vi "Begin.vi"() -> (0 "error out":errorcluster)   [LabVIEW 2012]
doc: "Called before other user functions, this VI is expected to open initial I/O refnums, load in file data, and do all program initialization. Notice that the <B>error out</B> terminal is simply used for data flow. Wiring it to other structures or subVIs ensures that this VI runs first."
uses:
  <vilib>/Rock Robotics/WPI/DriverStation/WPI_DriverStationRobotMode2.ctl
  <vilib>/Rock Robotics/WPI/Joystick/WPI_JoystickDeviceEnum.ctl
  <vilib>/Rock Robotics/WPI/Solenoid/WPI_SolenoidChannel.ctl
  <vilib>/Rock Robotics/SystemInterfaces/DIO/FPGA_DIORelayChannel.ctl
  <vilib>/Rock Robotics/WPI/Relay/WPI_RelayDirection.ctl
  <vilib>/Rock Robotics/SystemInterfaces/DIO/FPGA_DIOChannel.ctl
  <vilib>/Rock Robotics/WPI/Encoder/WPI_EncoderType.ctl
  <vilib>/Rock Robotics/SystemInterfaces/DIO/FPGA_DIOPWMChannel.ctl
  <vilib>/Rock Robotics/SystemInterfaces/AI/FPGA_AIGyroChannel.ctl
  <vilib>/Rock Robotics/SystemInterfaces/Typedef/FPGA_TypedefSolenoidModule.ctl
  Robot Global Data.vi
  <vilib>/Rock Robotics/WPI/Solenoid/WPI_SolenoidOpenSingle.vi
  <vilib>/Rock Robotics/WPI/Solenoid/Deprecated/WPI_SolenoidSetBool.vi
  <vilib>/Rock Robotics/WPI/Counter/WPI_CounterDigitalInputToDigitalSource.vi
  <vilib>/Rock Robotics/WPI/MotorControl/WPI_MotorControlOpen Jaguar.vi
  <vilib>/Rock Robotics/WPI/MotorControl/WPI_MotorControlOpen Victor.vi
  <vilib>/Rock Robotics/WPI/MotorControl/WPI_MotorControlOpen Talon.vi
  <vilib>/Rock Robotics/WPI/RobotDrive/WPI_RobotDriveOpen4MotorWithExistingMotors.vi
  <vilib>/Rock Robotics/WPI/Compressor/WPI_CompressorGetSetRefNum.vi
  <vilib>/Rock Robotics/SystemInterfaces/Typedef/FPGA_TypedefDigitalModule.ctl
  <vilib>/Rock Robotics/WPI/RobotDrive/WPI_RobotDriveOpen4MotorWithTalon.vi
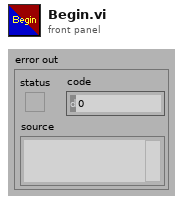
[diagram p1: front panel]
types:
  T1 = typedef "FPGA_DIOChannel.ctl" = enum8{"DIO 1", "DIO 2", "DIO 3", "DIO 4", "DIO 5", "DIO 6", "DIO 7", "DIO 8", "DIO 9", "DIO 10", "DIO 11", "DIO 12", "DIO 13", "DIO 14", "Invalid"}
  T2 = typedef "WPI_SolenoidChannel.ctl" = enum8{"Solenoid 1", "Solenoid 2", "Solenoid 3", "Solenoid 4", "Solenoid 5", "Solenoid 6", "Solenoid 7", "Solenoid 8", "Invalid"}
  T3 = typedef "FPGA_TypedefSolenoidModule.ctl" = enum16{"Solenoid Module 1", "Solenoid Module 2"}
  T4 = typedef "FPGA_AIGyroChannel.ctl" = enum8{"AI 1", "AI 2", "Invalid"}
  T5 = typedef "WPI_EncoderType.ctl" = enum16{"1x", "2x", "4x"}
  T6 = typedef "FPGA_DIORelayChannel.ctl" = enum8{"Relay 1", "Relay 2", "Relay 3", "Relay 4", "Relay 5", "Relay 6", "Relay 7", "Relay 8", "Invalid"}
  T7 = typedef "WPI_JoystickDeviceEnum.ctl" = enum16{"USB 1", "USB 2", "USB 3", "USB 4", "Kinect 1", "Kinect 2"}
  T8 = typedef "FPGA_DIOPWMChannel.ctl" = enum8{"PWM 1", "PWM 2", "PWM 3", "PWM 4", "PWM 5", "PWM 6", "PWM 7", "PWM 8", "PWM 9", "PWM 10", "Invalid"}
  T9 = typedef "WPI_RelayDirection.ctl" = enum16{"Both directions", "Forward only", "Reverse only"}
  T10 = typedef "WPI_DriverStationRobotMode2.ctl" = enum16{"Autonomous Disabled", "Autonomous Enabled", "Teleop Disabled", "Teleop Enabled", "Timeout", "Finish", "Test Disabled", "Test Enabled"}
  T11 = typedef "WPI_RobotDriveDevRef.ctl" = cluster{"DevStatus":errorcluster, "Motors[]":T12[], "Square Inputs":bool, "Max Output":dbl, "Isochronous":bool}
  T12 = typedef "WPI_MotorControlDeviceRef.ctl" = cluster{"DeviceStatus":errorcluster, "Type":enum16{"PWM", "CAN"}, "PWM":cluster{"Digital Module":T13, "PWM Channel":T8, "DeadBand":T14}, "CAN":cluster{"Device Number":u8, "Control Mode":T15, "Semaphore":T16, "Max Vout":dbl}, "Invert":bool, "TransformRef":T17, "InvTransformRef":T17}
  T13 = typedef "FPGA_TypedefDigitalModule.ctl" = enum16{"Digital Module 1", "Digital Module 2"}
  T14 = typedef "WPI_PWMDeadband.ctl" = cluster{"Name":string, "maxPositivePwm":i32, "minPositivePwm":i32, "centerPwm":i32, "maxNegativePwm":i32, "minNegativePwm":i32, "angularRange":u16}
  T15 = typedef "WPI_CANJaguar_ControlMode.ctl" = enum8{"Percent VBus", "Current", "Speed", "Position", "Voltage"}
  T16 = typedef "Semaphore RefNum" = refnum<k1>
  T17 = typedef "WPI_PWMTransform_ConPane.ctl" = refnum<vi>
  T18 = typedef "WPI_DigitalInputDevRef.ctl" = cluster{"DevStatus":errorcluster, "DIO Channel":T1, "Digital Module":T13}
  T19 = typedef "WPI_ServoDeviceRef.ctl" = cluster{"DeviceStatus":errorcluster, "Digital Module":T13, "PWM Channel":T8, "DeadBand":T14}
  T20 = typedef "WPI_CompressorDevRef.ctl" = cluster{"DevStatus":errorcluster, "DigitalInputDevRef":T18, "RelayDevRef":T21}
  T21 = typedef "WPI_RelayDevRef.ctl" = cluster{"DevStatus":errorcluster, "Relay Channel":T6, "Digital Module":T13, "Relay Direction":T9}
  T22 = typedef "WPI_JoystickDevRef.ctl" = cluster{"Device":T7}
  T23 = typedef "WPI_SolenoidDevRef.ctl" = cluster{"DevStatus":errorcluster, "Solenoid Module":T3, "Forward Solenoid Channel":T2, "Reverse Solenoid Channel":T2}
  T24 = typedef "FPGA_CounterEncoderSourceConvertionLVSourceType.ctl" = cluster{"DevStatus":errorcluster, "AnalogTriggerMode?":bool, "DigitalMode":cluster{"Digital Module":T13, "DIO Channel":T25}, "AnalogTriggerMode":cluster{"AnalogTriggerIndex":T26, "OutputType":T27}}
  T25 = typedef "FPGA_DIODigitalSourceChannel.ctl" = enum8{"DIO 1", "DIO 2", "DIO 3", "DIO 4", "DIO 5", "DIO 6", "DIO 7", "DIO 8", "DIO 9", "DIO 10", "DIO 11", "DIO 12", "DIO 13", "DIO 14", "Disabled"}
  T26 = typedef "FPGA_AnalogTriggerIndex.ctl" = enum8{"Trig 0", "Trig 1", "Trig 2", "Trig 3", "Trig 4", "Trig 5", "Trig 6", "Trig 7", "Invalid"}
  T27 = typedef "FPGA_AnalogTriggerOutType.ctl" = enum16{"InWindow", "TriggerState", "Rising", "Falling"}
  T28 = typedef "WPI_GyroDevRef.ctl" = cluster{"DevStatus":errorcluster, "Analog Module":T29, "Analog Channel":T30, "Offset":dbl, "Gain (VoltsPerDegree/Second)":dbl}
  T29 = typedef "FPGA_TypedefAnalogModule.ctl" = enum16{"Analog Module 1", "Analog Module 2"}
  T30 = typedef "FPGA_AIChannel.ctl" = enum8{"AI 1", "AI 2", "AI 3", "AI 4", "AI 5", "AI 6", "AI 7", "AI 8", "Invalid"}
  T31 = typedef "WPI_EncoderDevRef.ctl" = cluster{"DevStatus":errorcluster, "EncoderIndex":T32, "CounterIndex":T33, "DistancePerCount":dbl, "Decoding Type":T5}
  T32 = typedef "FPGA_EncoderIdx.ctl" = enum8{"Enc 0", "Enc 1", "Enc 2", "Enc 3", "Invalid"}
  T33 = typedef "FPGA_CounterCtrSystemIndex.ctl" = enum8{"Ctr 0", "Ctr 1", "Ctr 2", "Ctr 3", "Ctr 4", "Ctr 5", "Ctr 6", "Ctr 7", "Invalid"}
  T34 = cluster{"Target Voltage":dbl, "Target Speed":dbl, "Angle Up?":bool}
  T35 = cluster{"Target Voltage":dbl, "Target Speed":i32, "Angle Up?":bool}
  T36 = cluster{"Target Voltage":i32, "Target Speed":i32, "Angle Up?":bool}
  T37 = cluster{"Target Voltage":dbl, "Target Speed":i32, "Angle Up?":bool}[]
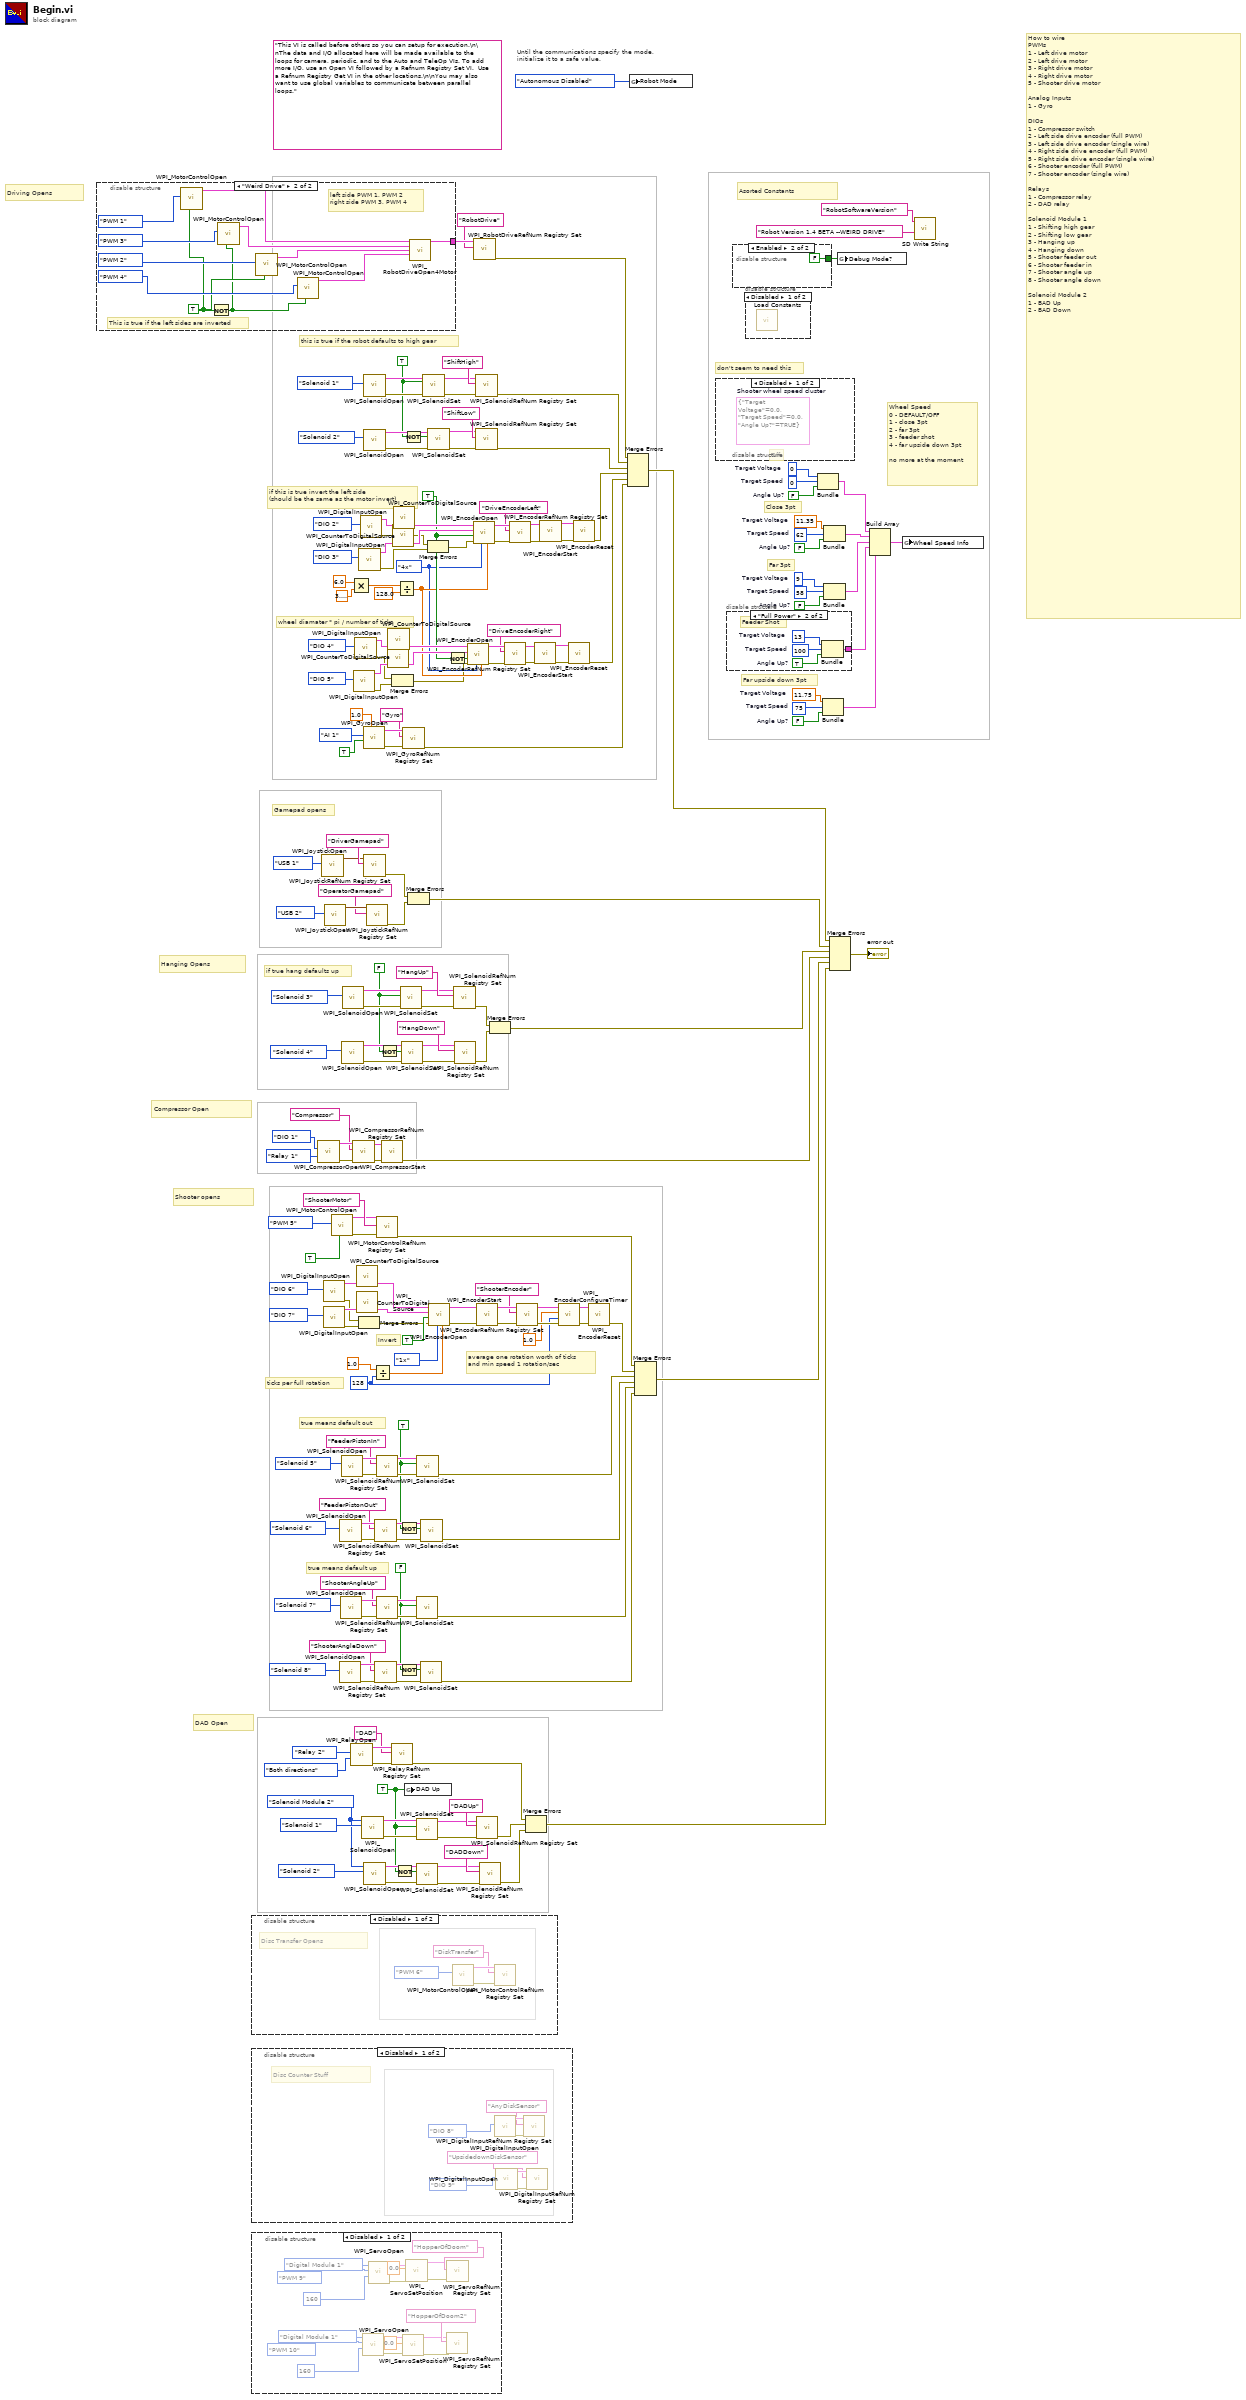
[diagram p0: block diagram]
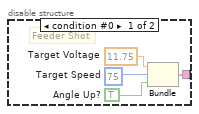
[diagram p3: hidden frame]
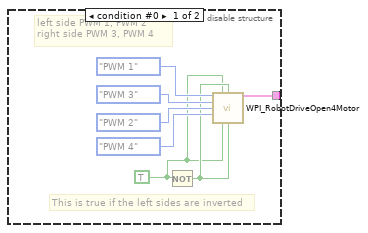
[diagram p4: hidden frame]
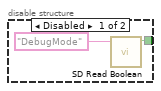
[diagram p5: hidden frame]
diagram:
  w3 = FALSE  # Angle Up?
  w2 = 58  # Target Speed
  w1 = 9  # Target Voltage
  w7 = FALSE  # Angle Up?
  w6 = 75  # Target Speed
  w5 = 11.75  # Target Voltage
  w11 = FALSE  # Angle Up?
  w10 = 0  # Target Speed
  w9 = 0  # Target Voltage
  w13 = u8 128 ("Number Samples to Average")
  w20 = FALSE  # Angle Up?
  w21 = 62  # Target Speed
  w22 = 11.35  # Target Voltage
  w82 = FALSE
  w96 = TRUE
  w57 = TRUE
  w59 = FPGA_TypedefSolenoidModule."Solenoid Module 2" ("Solenoid Module (Module 1)")
  w60 = FALSE
  w62 = WPI_EncoderType."4x" ("Decoding Type")
  w64 = TRUE ("Invert Direction (False)")
  w80 = TRUE
  (unwired) "This VI is called before others so you can setup for execution.\n\nThe data and I/O allocated here will be made available to the loops for camera, periodic, and to the Auto and TeleOp VIs. To add more I/O, use an Open VI followed by a Refnum Registry Set VI.  Use a Refnum Registry Get VI in the other locations.\n\nYou may also want to use global variables to communicate between parallel loops."
  # "don't seem to need this"
  # "Far 3pt"
  # "Far upside down 3pt"
  # "average one rotation worth of ticks\nand min speed 1 rotation/sec"
  # "Close 3pt"
  # "How to wire\nPWMs\n1 - Left drive motor\n2 - Left drive motor\n3 - Right drive motor\n4 - Right drive motor\n5 - Shooter drive motor\n\nAnalog Inputs\n1 - Gyro\n\nDIOs\n1 - Compressor switch\n2 - Left side drive encoder (full PWM)\n3 - Left side drive encoder (single wire)\n4 - Right side drive encoder (full PWM)\n5 - Right side drive encoder (single wire)\n6 - Shooter encoder (full PWM)\n7 - Shooter encoder (single wire)\n\nRelays\n1 - Compressor relay\n2 - DAD relay\n\nSolenoid Module 1\n1 - Shifting high gear\n2 - Shifting low gear\n3 - Hanging up\n4 - Hanging down\n5 - Shooter feeder out\n6 - Shooter feeder in\n7 - Shooter angle up\n8 - Shooter angle down\n\nSolenoid Module 2\n1 - BAD Up\n2 - BAD Down"
  # "Asorted Constants"
  # "true means default up"
  # "true means default out"
  # "if true hang defaults up"
  # "Gamepad opens"
  # "wheel diamater * pi / number of ticks"
  # "if this is true invert the left side\n(should be the same as the motor invert)"
  # "this is true if the robot defaults to high gear"
  # "Compressor Open"
  # "Wheel Speed\n0 - DEFAULT/OFF\n1 - close 3pt\n2 - far 3pt\n3 - feeder shot\n4 - far upside down 3pt\n\nno more at the moment"
  # "DAD Open"
  # "Hanging Opens"
  # "Driving Opens"
  # "Shooter opens"
  # "Invert"
  # "ticks per full rotation"
  # "Until the communications specify the mode,\ninitialize it to a safe value."
  n1 = disable-structure shown="\"Weird Drive\"" {
    disable-tunnel: [w217 w232] -> w210
    frame condition #0 {
      w215 = TRUE ("Rear Left Motor Inverted")
      # "left side PWM 1, PWM 2\nright side PWM 3, PWM 4"
      # "This is true if the left sides are inverted"
      n2 = Not(x=w215) -> (.not. x?=w216:bool)
      n3 = call-poly <vilib>:"WPI_RobotDriveOpen4Motor.vi"("Rear Left Motor"=FPGA_DIOPWMChannel."PWM 1", "Rear Left Motor Inverted"=w215, "Rear Right Motor Inverted"=w216, "Rear Right Motor"=FPGA_DIOPWMChannel."PWM 3", "Front Left Motor"=FPGA_DIOPWMChannel."PWM 2", "Front Right Motor"=FPGA_DIOPWMChannel."PWM 4" ("Front Left Motor"), "Front Left Motor Inverted"=w215, "Front Right Motor Inverted"=w216) -> ("RobotDriveDevRef"=w217:T11)  [unwired: 6 in, 1 out]
    }
    frame condition #1 (active) {
      w227 = TRUE ("Rear Left Motor Inverted")
      # "left side PWM 1, PWM 2\nright side PWM 3, PWM 4"
      # "This is true if the left sides are inverted"
      n4 = call-poly <vilib>:"WPI_MotorControlOpen.vi"("Invert"=w227, "PWM Channel"=FPGA_DIOPWMChannel."PWM 1" ("Rear Left Motor")) -> ("MotorControlDeviceRef"=w225:T12)  [unwired: 8 in, 1 out]
      n5 = Not(x=w227) -> (.not. x?=w226:bool)
      n6 = call-poly <vilib>:"WPI_MotorControlOpen.vi"("Invert"=w226, "PWM Channel"=FPGA_DIOPWMChannel."PWM 3" ("Rear Right Motor")) -> ("MotorControlDeviceRef"=w224:T12)  [unwired: 8 in, 1 out]
      n7 = call-poly <vilib>:"WPI_MotorControlOpen.vi"("Invert"=w227, "PWM Channel"=FPGA_DIOPWMChannel."PWM 2" ("Front Left Motor")) -> ("MotorControlDeviceRef"=w223:T12)  [unwired: 8 in, 1 out]
      n8 = call-poly <vilib>:"WPI_MotorControlOpen.vi"("Invert"=w226, "PWM Channel"=FPGA_DIOPWMChannel."PWM 4" ("Front Left Motor")) -> ("MotorControlDeviceRef"=w222:T12)  [unwired: 8 in, 1 out]
      n9 = call-poly <vilib>:"WPI_RobotDriveOpen4Motor.vi"("Rear Left Motor Dev Ref"=w225, "Rear Right Motor Dev Ref"=w224, "Front Left Motor Dev Ref"=w223, "Front Right Motor Dev Ref"=w222) -> ("RobotDriveDevRef"=w232:T11)  [unwired: 10 in, 1 out]
    }
  }
  n10 = disable-structure shown="Disabled" {
    frame Disabled {
      # "Disc Transfer Opens"
      n11 = call-poly <vilib>:"WPI_MotorControlOpen.vi"("PWM Channel"=FPGA_DIOPWMChannel."PWM 6") -> ("error out"=w234:errorcluster, "MotorControlDeviceRef"=w235:T12)  [unwired: 9 in]
      n12 = call <vilib>:"WPI_MotorControlRefNum Registry Set.vi"("error in (no error)"=w234, "refnum name"="DiskTransfer", "MotorControlDevRef"=w235) -> ()  [unwired: 7 in, 2 out]
    }
    frame Enabled {
    }
  }
  n13 = disable-structure shown="Disabled" {
    frame Disabled {
      # "Disc Counter Stuff"
      n14 = call <vilib>:"WPI_DigitalInputOpen.vi"("DIO Channel"=FPGA_DIOChannel."DIO 8") -> ("error out"=w244:errorcluster, "DigitalInputDevRef"=w243:T18)  [unwired: 9 in]
      n15 = call <vilib>:"WPI_DigitalInputOpen.vi"("DIO Channel"=FPGA_DIOChannel."DIO 9") -> ("error out"=w242:errorcluster, "DigitalInputDevRef"=w241:T18)  [unwired: 9 in]
      n16 = call <vilib>:"WPI_DigitalInputRefNum Registry Set.vi"("error in (no error)"=w244, "refnum name"="AnyDiskSensor", "DigitalInputDevRef"=w243) -> ()  [unwired: 7 in, 2 out]
      n17 = call <vilib>:"WPI_DigitalInputRefNum Registry Set.vi"("error in (no error)"=w242, "refnum name"="UpsidedownDiskSensor", "DigitalInputDevRef"=w241) -> ()  [unwired: 7 in, 2 out]
    }
    frame Enabled {
    }
  }
  n18 = disable-structure shown="Disabled" {
    frame Disabled {
      n19 = call <vilib>:"WPI_ServoOpen.vi"("Angular Range"=160, "PWM Channel"=FPGA_DIOPWMChannel."PWM 10", "Digital Module (Module 1)"=FPGA_TypedefDigitalModule."Digital Module 1") -> ("error out"=w250:errorcluster, "ServoDeviceRef"=w249:T19)  [unwired: 7 in]
      n20 = call <vilib>:"WPI_ServoOpen.vi"("Angular Range"=160, "PWM Channel"=FPGA_DIOPWMChannel."PWM 9", "Digital Module (Module 1)"=FPGA_TypedefDigitalModule."Digital Module 1") -> ("error out"=w254:errorcluster, "ServoDeviceRef"=w253:T19)  [unwired: 7 in]
      n21 = call <vilib>:"WPI_ServoSetPosition.vi"("error in (no error)"=w250, "Position"=0.0, "ServoDeviceRef"=w249) -> ("error out"=w247:errorcluster, "ServoDeviceRef"=w248:T19)  [unwired: 7 in]
      n22 = call <vilib>:"WPI_ServoSetPosition.vi"("error in (no error)"=w254, "Position"=0.0, "ServoDeviceRef"=w253) -> ("error out"=w252:errorcluster, "ServoDeviceRef"=w251:T19)  [unwired: 7 in]
      n23 = call <vilib>:"WPI_ServoRefNum Registry Set.vi"("error in (no error)"=w247, "refnum name"="HopperOfDoom2", "ServoDeviceRef"=w248) -> ()  [unwired: 7 in, 2 out]
      n24 = call <vilib>:"WPI_ServoRefNum Registry Set.vi"("error in (no error)"=w252, "refnum name"="HopperOfDoom", "ServoDeviceRef"=w251) -> ()  [unwired: 7 in, 2 out]
    }
    frame Enabled {
    }
  }
  n25 = call <vilib>:"WPI_CompressorOpen.vi"("Pressure Switch DIO Channel"=FPGA_DIOChannel."DIO 1", "Relay Channel"=FPGA_DIORelayChannel."Relay 1") -> ("CompressorDevRef"=w162:T20, "error out"=w160:errorcluster)  [unwired: 12 in]
  n26 = call <vilib>:"WPI_JoystickOpen.vi"("JoystickDevice"=WPI_JoystickDeviceEnum."USB 1") -> ("JoystickDevRef"=w212:T22)  [unwired: 10 in]
  n27 = call <vilib>:"WPI_DigitalInputOpen.vi"("DIO Channel"=FPGA_DIOChannel."DIO 6") -> ("error out"=w178:errorcluster, "DigitalInputDevRef"=w191:T18)  [unwired: 9 in]
  n28 = call <vilib>:"WPI_DigitalInputOpen.vi"("DIO Channel"=FPGA_DIOChannel."DIO 7") -> ("error out"=w177:errorcluster, "DigitalInputDevRef"=w187:T18)  [unwired: 9 in]
  n29 = call <vilib>:"WPI_JoystickOpen.vi"("JoystickDevice"=WPI_JoystickDeviceEnum."USB 2") -> ("JoystickDevRef"=w164:T22)  [unwired: 10 in]
  n30 = call-poly <vilib>:"WPI_MotorControlOpen.vi"("Invert"=TRUE, "PWM Channel"=FPGA_DIOPWMChannel."PWM 5") -> ("error out"=w171:errorcluster, "MotorControlDeviceRef"=w172:T12)  [unwired: 8 in]
  n31 = call-poly <vilib>:"WPI_SolenoidOpen.vi"("Solenoid Channel"=WPI_SolenoidChannel."Solenoid 8") -> ("error out"=w92:errorcluster, "SolenoidDevRef"=w91:T23)  [unwired: 9 in]
  n32 = call-poly <vilib>:"WPI_SolenoidOpen.vi"("Solenoid Channel"=WPI_SolenoidChannel."Solenoid 6") -> ("error out"=w106:errorcluster, "SolenoidDevRef"=w105:T23)  [unwired: 9 in]
  n33 = call-poly <vilib>:"WPI_SolenoidOpen.vi"("Solenoid Channel"=WPI_SolenoidChannel."Solenoid 7") -> ("error out"=w87:errorcluster, "SolenoidDevRef"=w88:T23)  [unwired: 9 in]
  n34 = call-poly <vilib>:"WPI_SolenoidOpen.vi"("Solenoid Channel"=WPI_SolenoidChannel."Solenoid 5") -> ("error out"=w101:errorcluster, "SolenoidDevRef"=w102:T23)  [unwired: 9 in]
  n35 = call-poly <vilib>:"WPI_SolenoidOpen.vi"("Solenoid Channel"=WPI_SolenoidChannel."Solenoid 4") -> ("error out"=w128:errorcluster, "SolenoidDevRef"=w129:T23)  [unwired: 9 in]
  n36 = call-poly <vilib>:"WPI_SolenoidOpen.vi"("Solenoid Channel"=WPI_SolenoidChannel."Solenoid 3") -> ("error out"=w131:errorcluster, "SolenoidDevRef"=w130:T23)  [unwired: 9 in]
  n37 = Multiply(x=6.0, y=3.141592653589793) -> (x*y=w149:dbl)
  n38 = call <vilib>:"WPI_RelayOpen.vi"("Relay Direction"=WPI_RelayDirection."Both directions", "Relay Channel"=FPGA_DIORelayChannel."Relay 2") -> ("error out"=w194:errorcluster, "RelayDevRef"=w193:T21)  [unwired: 8 in]
  n39 = call <vilib>:"WPI_CompressorRefNum Registry Set.vi"("error in (no error)"=w160, "refnum name"="Compressor", "CompressorDevRef"=w162) -> ("error out"=w110:errorcluster, "CompressorDevRef"=w111:T20)  [unwired: 7 in]
  n40 = call <vilib>:"WPI_DigitalInputOpen.vi"("DIO Channel"=FPGA_DIOChannel."DIO 5") -> ("error out"=w50:errorcluster, "DigitalInputDevRef"=w72:T18)  [unwired: 9 in]
  n41 = call <vilib>:"WPI_DigitalInputOpen.vi"("DIO Channel"=FPGA_DIOChannel."DIO 4") -> ("error out"=w49:errorcluster, "DigitalInputDevRef"=w71:T18)  [unwired: 9 in]
  n42 = call-poly <vilib>:"WPI_CounterToDigitalSource.vi"("DigitalInputDevRef"=w191) -> ("Digital Source"=w190:T24)  [unwired: 6 in]
  n43 = call-poly <vilib>:"WPI_CounterToDigitalSource.vi"("DigitalInputDevRef"=w187) -> ("Digital Source"=w184:T24)  [unwired: 6 in]
  n44 = Merge Errors(w178, w177) -> (w179:errorcluster)
  n45 = call <vilib>:"WPI_DigitalInputOpen.vi"("DIO Channel"=FPGA_DIOChannel."DIO 3") -> ("error out"=w45:errorcluster, "DigitalInputDevRef"=w152:T18)  [unwired: 9 in]
  n46 = call <vilib>:"WPI_DigitalInputOpen.vi"("DIO Channel"=FPGA_DIOChannel."DIO 2") -> ("error out"=w46:errorcluster, "DigitalInputDevRef"=w153:T18)  [unwired: 9 in]
  n47 = call-poly <vilib>:"WPI_SolenoidOpen.vi"("Solenoid Channel"=WPI_SolenoidChannel."Solenoid 1", "Solenoid Module (Module 1)"=w59) -> ("error out"=w115:errorcluster, "SolenoidDevRef"=w119:T23)  [unwired: 8 in]
  n48 = call <vilib>:"WPI_GyroOpen.vi"("Calibration Time (s)"=1.0, "Calibrate On Open"=TRUE, "Analog Channel"=FPGA_AIGyroChannel."AI 1") -> ("error out"=w141:errorcluster, "GyroDevRef"=w140:T28)  [unwired: 6 in, 1 out]
  n49 = call-poly <vilib>:"WPI_SolenoidOpen.vi"("Solenoid Channel"=WPI_SolenoidChannel."Solenoid 1") -> ("error out"=w201:errorcluster, "SolenoidDevRef"=w204:T23)  [unwired: 9 in]
  n50 = call-poly <vilib>:"WPI_SolenoidOpen.vi"("Solenoid Channel"=WPI_SolenoidChannel."Solenoid 2") -> ("error out"=w198:errorcluster, "SolenoidDevRef"=w200:T23)  [unwired: 9 in]
  n51 = call <vilib>:"WPI_JoystickRefNum Registry Set.vi"("refnum name"="DriverGamepad", "JoystickDevRef"=w212) -> ("error out"=w42:errorcluster)  [unwired: 8 in, 1 out]
  n52 = call-poly <vilib>:"WPI_SolenoidOpen.vi"("Solenoid Channel"=WPI_SolenoidChannel."Solenoid 2", "Solenoid Module (Module 1)"=w59) -> ("error out"=w112:errorcluster, "SolenoidDevRef"=w117:T23)  [unwired: 8 in]
  n53 = call <vilib>:"WPI_JoystickRefNum Registry Set.vi"("refnum name"="OperatorGamepad", "JoystickDevRef"=w164) -> ("error out"=w41:errorcluster)  [unwired: 8 in, 1 out]
  n54 = Divide(x=1.0, y=w13) -> (x/y=w14:dbl)
  n55 = call <vilib>:"WPI_SolenoidRefNum Registry Set.vi"("error in (no error)"=w106, "refnum name"="FeederPistonOut", "SolenoidDevRef"=w105) -> ("error out"=w108:errorcluster, "SolenoidDevRef"=w107:T23)  [unwired: 7 in]
  n56 = call <vilib>:"WPI_SolenoidRefNum Registry Set.vi"("error in (no error)"=w92, "refnum name"="ShooterAngleDown", "SolenoidDevRef"=w91) -> ("error out"=w94:errorcluster, "SolenoidDevRef"=w93:T23)  [unwired: 7 in]
  n57 = call <vilib>:"WPI_MotorControlRefNum Registry Set.vi"("error in (no error)"=w171, "refnum name"="ShooterMotor", "MotorControlDevRef"=w172) -> ("error out"=w38:errorcluster)  [unwired: 7 in, 1 out]
  n58 = call <vilib>:"WPI_SolenoidRefNum Registry Set.vi"("error in (no error)"=w101, "refnum name"="FeederPistonIn", "SolenoidDevRef"=w102) -> ("error out"=w99:errorcluster, "SolenoidDevRef"=w100:T23)  [unwired: 7 in]
  n59 = call <vilib>:"WPI_SolenoidRefNum Registry Set.vi"("error in (no error)"=w87, "refnum name"="ShooterAngleUp", "SolenoidDevRef"=w88) -> ("error out"=w85:errorcluster, "SolenoidDevRef"=w86:T23)  [unwired: 7 in]
  n60 = Not(x=w60) -> (.not. x?=w61:bool)
  n61 = call <vilib>:"WPI_CompressorStart.vi"("error in (no error)"=w110, "CompressorDevRef"=w111) -> ("error out"=w26:errorcluster)  [unwired: 8 in, 1 out]
  n62 = call-poly <vilib>:"WPI_CounterToDigitalSource.vi"("DigitalInputDevRef"=w72) -> ("Digital Source"=w69:T24)  [unwired: 6 in]
  n63 = call-poly <vilib>:"WPI_CounterToDigitalSource.vi"("DigitalInputDevRef"=w71) -> ("Digital Source"=w67:T24)  [unwired: 6 in]
  n64 = call <vilib>:"WPI_RelayRefNum Registry Set.vi"("error in (no error)"=w194, "refnum name"="DAD", "RelayDevRef"=w193) -> ("error out"=w32:errorcluster)  [unwired: 7 in, 1 out]
  n65 = Merge Errors(w49, w50) -> (w48:errorcluster)
  n66 = call-poly <vilib>:"WPI_CounterToDigitalSource.vi"("DigitalInputDevRef"=w152) -> ("Digital Source"=w155:T24)  [unwired: 6 in]
  n67 = call-poly <vilib>:"WPI_CounterToDigitalSource.vi"("DigitalInputDevRef"=w153) -> ("Digital Source"=w157:T24)  [unwired: 6 in]
  n68 = Not(x=w57) -> (.not. x?=w58:bool)
  n69 = Divide(x=w149, y=128.0 ("x")) -> (x/y=w63:dbl)
  n70 = Not(x=w82) -> (.not. x?=w95:bool)
  n71 = Not(x=w96) -> (.not. x?=w109:bool)
  n72 = call-poly <vilib>:"WPI_SolenoidSet.vi"("error in (no error)"=w131, "Value"=w60, "SolenoidDevRef"=w130) -> ("error out"=w124:errorcluster, "SolenoidDevRef"=w127:T23)  [unwired: 7 in]
  n73 = call-poly <vilib>:"WPI_SolenoidSet.vi"("error in (no error)"=w128, "Value"=w61, "SolenoidDevRef"=w129) -> ("error out"=w125:errorcluster, "SolenoidDevRef"=w126:T23)  [unwired: 7 in]
  n74 = Not(x=w80) -> (.not. x?=w81:bool)
  n75 = call <vilib>:"WPI_GyroRefNum Registry Set.vi"("error in (no error)"=w141, "refnum name"="Gyro", "GyroDevRef"=w140) -> ("error out"=w43:errorcluster)  [unwired: 7 in, 1 out]
  n76 = global write "Robot Global Data.vi" "DAD Up"(w57) -> ()
  n77 = Merge Errors(w42, w41) -> (w28:errorcluster)
  n78 = call-poly <vilib>:"WPI_SolenoidSet.vi"("error in (no error)"=w85, "Value"=w82, "SolenoidDevRef"=w86) -> ("error out"=w34:errorcluster)  [unwired: 7 in, 1 out]
  n79 = call-poly <vilib>:"WPI_SolenoidSet.vi"("error in (no error)"=w115, "Value"=w57, "SolenoidDevRef"=w119) -> ("error out"=w114:errorcluster, "SolenoidDevRef"=w118:T23)  [unwired: 7 in]
  n80 = call-poly <vilib>:"WPI_SolenoidSet.vi"("error in (no error)"=w112, "Value"=w58, "SolenoidDevRef"=w117) -> ("error out"=w113:errorcluster, "SolenoidDevRef"=w116:T23)  [unwired: 7 in]
  n81 = call-poly <vilib>:"WPI_SolenoidSet.vi"("error in (no error)"=w99, "Value"=w96, "SolenoidDevRef"=w100) -> ("error out"=w36:errorcluster)  [unwired: 7 in, 1 out]
  n82 = call-poly <vilib>:"WPI_SolenoidSet.vi"("error in (no error)"=w94, "Value"=w95, "SolenoidDevRef"=w93) -> ("error out"=w33:errorcluster)  [unwired: 7 in, 1 out]
  n83 = call-poly <vilib>:"WPI_SolenoidSet.vi"("error in (no error)"=w108, "Value"=w109, "SolenoidDevRef"=w107) -> ("error out"=w35:errorcluster)  [unwired: 7 in, 1 out]
  n84 = call-poly <vilib>:"WPI_SolenoidSet.vi"("error in (no error)"=w201, "Value"=w80, "SolenoidDevRef"=w204) -> ("error out"=w202:errorcluster, "SolenoidDevRef"=w203:T23)  [unwired: 7 in]
  n85 = Merge Errors(w46, w45) -> (w47:errorcluster)
  n86 = call-poly <vilib>:"WPI_SolenoidSet.vi"("error in (no error)"=w198, "Value"=w81, "SolenoidDevRef"=w200) -> ("error out"=w197:errorcluster, "SolenoidDevRef"=w199:T23)  [unwired: 7 in]
  n87 = call <vilib>:"WPI_EncoderOpen.vi"("DistancePerCount"=w14, "Decoding Type"=WPI_EncoderType."1x", "error in (no error)"=w179, "Invert Direction (False)"=TRUE, "BSource"=w184, "ASource"=w190) -> ("error out"=w180:errorcluster, "EncoderDevRef"=w181:T31)  [unwired: 4 in]
  n88 = Not(x=w64) -> (.not. x?=w65:bool)
  n89 = call <vilib>:"WPI_SolenoidRefNum Registry Set.vi"("error in (no error)"=w124, "refnum name"="HangUp", "SolenoidDevRef"=w127) -> ("error out"=w40:errorcluster)  [unwired: 7 in, 1 out]
  n90 = call <vilib>:"WPI_SolenoidRefNum Registry Set.vi"("error in (no error)"=w125, "refnum name"="HangDown", "SolenoidDevRef"=w126) -> ("error out"=w39:errorcluster)  [unwired: 7 in, 1 out]
  n91 = call <vilib>:"WPI_EncoderOpen.vi"("DistancePerCount"=w63, "Decoding Type"=w62, "error in (no error)"=w48, "Invert Direction (False)"=w65, "BSource"=w69, "ASource"=w67) -> ("error out"=w73:errorcluster, "EncoderDevRef"=w74:T31)  [unwired: 4 in]
  n92 = call <vilib>:"WPI_EncoderOpen.vi"("DistancePerCount"=w63, "Decoding Type"=w62, "error in (no error)"=w47, "Invert Direction (False)"=w64, "BSource"=w155, "ASource"=w157) -> ("error out"=w148:errorcluster, "EncoderDevRef"=w147:T31)  [unwired: 4 in]
  n93 = call <vilib>:"WPI_RobotDriveRefNum Registry Set.vi"("refnum name"="RobotDrive", "RobotDriveDevRef"=w210) -> ("error out"=w54:errorcluster)  [unwired: 8 in, 1 out]
  n94 = call <vilib>:"WPI_SolenoidRefNum Registry Set.vi"("error in (no error)"=w202, "refnum name"="ShiftHigh", "SolenoidDevRef"=w203) -> ("error out"=w53:errorcluster)  [unwired: 7 in, 1 out]
  n95 = call <vilib>:"WPI_SolenoidRefNum Registry Set.vi"("error in (no error)"=w197, "refnum name"="ShiftLow", "SolenoidDevRef"=w199) -> ("error out"=w52:errorcluster)  [unwired: 7 in, 1 out]
  n96 = call <vilib>:"WPI_EncoderStart.vi"("error in (no error)"=w180, "EncoderDevRef"=w181) -> ("error out"=w176:errorcluster, "EncoderDevRef"=w182:T31)  [unwired: 8 in]
  n97 = call <vilib>:"WPI_SolenoidRefNum Registry Set.vi"("error in (no error)"=w114, "refnum name"="DADUp", "SolenoidDevRef"=w118) -> ("error out"=w31:errorcluster)  [unwired: 7 in, 1 out]
  n98 = call <vilib>:"WPI_SolenoidRefNum Registry Set.vi"("error in (no error)"=w113, "refnum name"="DADDown", "SolenoidDevRef"=w116) -> ("error out"=w30:errorcluster)  [unwired: 7 in, 1 out]
  n99 = Merge Errors(w40, w39) -> (w27:errorcluster)
  n100 = call <vilib>:"WPI_EncoderRefNum Registry Set.vi"("error in (no error)"=w73, "refnum name"="DriveEncoderRight", "EncoderDevRef"=w74) -> ("error out"=w75:errorcluster, "EncoderDevRef"=w76:T31)  [unwired: 7 in]
  n101 = call <vilib>:"WPI_EncoderRefNum Registry Set.vi"("error in (no error)"=w148, "refnum name"="DriveEncoderLeft", "EncoderDevRef"=w147) -> ("error out"=w146:errorcluster, "EncoderDevRef"=w145:T31)  [unwired: 7 in]
  n102 = call <vilib>:"WPI_EncoderRefNum Registry Set.vi"("error in (no error)"=w176, "refnum name"="ShooterEncoder", "EncoderDevRef"=w182) -> ("error out"=w167:errorcluster, "EncoderDevRef"=w168:T31)  [unwired: 7 in]
  n103 = Merge Errors(w32, w31, w30) -> (w24:errorcluster)
  n104 = call <vilib>:"WPI_EncoderStart.vi"("error in (no error)"=w75, "EncoderDevRef"=w76) -> ("error out"=w77:errorcluster, "EncoderDevRef"=w78:T31)  [unwired: 8 in]
  n105 = call <vilib>:"WPI_EncoderStart.vi"("error in (no error)"=w146, "EncoderDevRef"=w145) -> ("error out"=w144:errorcluster, "EncoderDevRef"=w143:T31)  [unwired: 8 in]
  n106 = call <vilib>:"WPI_EncoderConfigureTimer.vi"("error in (no error)"=w167, "Number Samples to Average"=w13, "Minimum Rate"=1.0, "EncoderDevRef"=w168) -> ("error out"=w170:errorcluster, "EncoderDevRef"=w169:T31)  [unwired: 6 in]
  n107 = call <vilib>:"WPI_EncoderReset.vi"("error in (no error)"=w77, "EncoderDevRef"=w78) -> ("error out"=w44:errorcluster)  [unwired: 8 in, 1 out]
  n108 = call <vilib>:"WPI_EncoderReset.vi"("error in (no error)"=w144, "EncoderDevRef"=w143) -> ("error out"=w51:errorcluster)  [unwired: 8 in, 1 out]
  n109 = call <vilib>:"WPI_EncoderReset.vi"("error in (no error)"=w170, "EncoderDevRef"=w169) -> ("error out"=w37:errorcluster)  [unwired: 8 in, 1 out]
  n110 = Merge Errors(w54, w53, w52, w51, w44, w43) -> (w29:errorcluster)
  n111 = global write "Robot Global Data.vi" "Robot Mode"(WPI_DriverStationRobotMode2."Autonomous Disabled" ("Robot Mode")) -> ()
  n112 = Merge Errors(w38, w37, w36, w35, w34, w33) -> (w25:errorcluster)
  n113 = disable-structure shown="Disabled" {
    frame Disabled {
      (unwired) T34 {"Target Voltage"=0.0, "Target Speed"=0.0, "Angle Up?"=TRUE}  # Shooter wheel speed cluster
      # "Off"
    }
    frame Enabled {
    }
  }
  n114 = disable-structure shown="\"Full Power\"" {
    disable-tunnel: [w263 w267] -> w17
    frame condition #0 {
      w264 = TRUE  # Angle Up?
      w265 = 75  # Target Speed
      w266 = 11.75  # Target Voltage
      # "Feeder Shot"
      n115 = Bundle("Target Voltage"=w266, "Target Speed"=w265, "Angle Up?"=w264) -> (w263:T35)  [unwired: 1 in]
    }
    frame condition #1 (active) {
      w268 = TRUE  # Angle Up?
      w269 = 100  # Target Speed
      w270 = 13  # Target Voltage
      # "Feeder Shot"
      n116 = Bundle("Target Voltage"=w270, "Target Speed"=w269, "Angle Up?"=w268) -> (w267:T36)  [unwired: 1 in]
    }
  }
  n117 = disable-structure shown="Enabled" {
    disable-tunnel: [w271 FALSE ("Debug Mode?")] -> w15
    frame Disabled {
      n118 = call <vilib>:"SD Read Boolean.vi"("Name"="DebugMode") -> ("Boolean"=w271:bool)  [unwired: 8 in, 2 out]
    }
    frame Enabled {
    }
  }
  n119 = disable-structure shown="Disabled" {
    frame Disabled {
      n120 = call "Load Constants.vi"() -> ()  [unwired: 12 in]
    }
    frame Enabled {
    }
  }
  n121 = Bundle("Target Voltage"=w9, "Target Speed"=w10, "Angle Up?"=w11) -> (w8:T36)  [unwired: 1 in]
  n122 = Bundle("Target Voltage"=w5, "Target Speed"=w6, "Angle Up?"=w7) -> (w4:T35)  [unwired: 1 in]
  n123 = Bundle("Target Voltage"=w22, "Target Speed"=w21, "Angle Up?"=w20) -> (w19:T35)  [unwired: 1 in]
  n124 = Bundle("Target Voltage"=w1, "Target Speed"=w2, "Angle Up?"=w3) -> (w18:T36)  [unwired: 1 in]
  n125 = Merge Errors(w29, w28, w27, w26, w25, w24) -> (→"error out":errorcluster)
  n126 = global write "Robot Global Data.vi" "Debug Mode?"(w15) -> ()
  n127 = Build Array(w8, w19, w18, w17, w4) -> (w16:T37)
  n128 = global write "Robot Global Data.vi" "Wheel Speed Info"(w16) -> ()
  n129 = call <vilib>:"SD Write String.vi"("String"="Robot Version 1.4 BETA --WEIRD DRIVE", "Name"="RobotSoftwareVersion") -> ()  [unwired: 8 in, 2 out]
